vi "2Dstart_BD_ver10_two_daqs.vi"(0 "Master Ctr (Ctr0)":tag, 1 "Master Ctr Terminal (PFI0)":tag, 2 "Galvo Hardware":T2, 3 "Camera Hardware":T1, 4 "input cluster":T4, 5 "error in (no error)":errorcluster, 6 "B-Scan Frequency":dbl=100.0, 7 "A-scans per Image":u32, 8 "Camera Delay (us)":dbl format="%.6f", 9 "A-scans per Cross Section":u32, 11 "Galvo Trigg per Cross Section":u32) -> (13 "Image Size":u32, 14 "Master Ctr Task Out":refnum<k21>, 15 "Galvo AO Task Out":refnum<k21>, 16 "Camera Ctr Task Out":refnum<k21>, 17 "Galvo Ctr Task Out":refnum<k21>, 18 "output cluster for DLL":T3, 19 "AO Err Out":errorcluster)   [LabVIEW 2017]
uses:
  <vilib>/DAQmx/write.llb/DAQmx Write (Analog 2D DBL NChan NSamp).vi
  <vilib>/DAQmx/create/channels.llb/DAQmx Create Channel (CO-Pulse Generation-Frequency).vi
  <vilib>/DAQmx/configure/timing.llb/DAQmx Timing (Implicit).vi
  <vilib>/DAQmx/configure/trigger.llb/DAQmx Start Trigger (Digital Edge).vi
  <vilib>/DAQmx/create/channels.llb/DAQmx Create Channel (AO-Voltage-Basic).vi
  <vilib>/DAQmx/configure/timing.llb/DAQmx Timing (Sample Clock).vi
  <vilib>/DAQmx/miscellaneous.llb/DAQmx Fill In Error Info.vi
  <resource>/objmgr/daqmx.rc
panel:
  out "B-Scan Frequency 2":dbl
  in  "counter":tag
  out "error out":errorcluster
  out "task out":refnum<k21>
  in  "2D frequency":i16
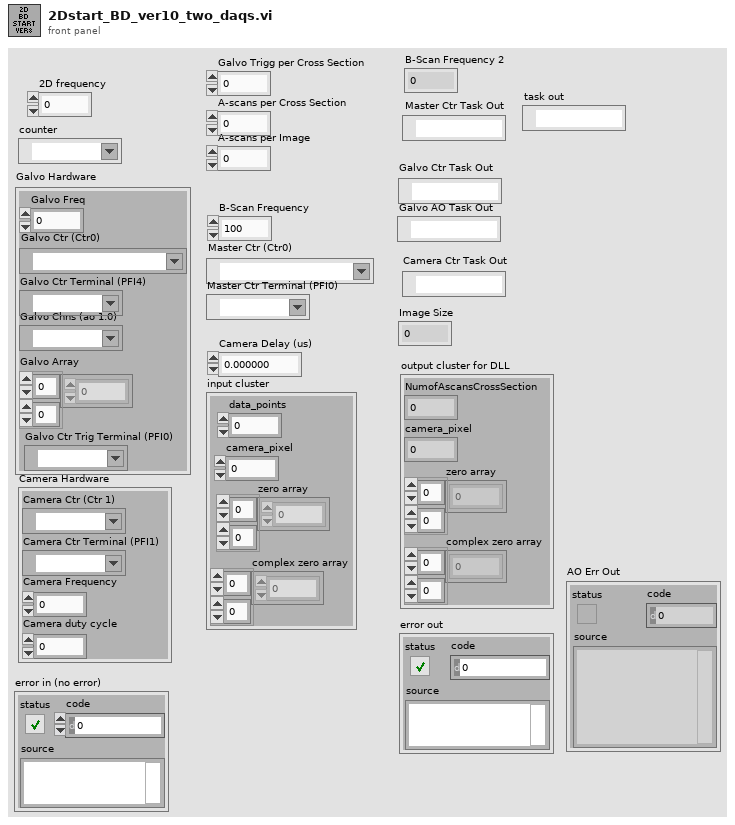
[diagram p1: front panel]
types:
  T1 = cluster{"Camera Ctr (Ctr 1)":tag, "Camera Ctr Terminal (PFI1)":tag, "Camera Frequency":dbl, "Camera duty cycle":dbl}
  T2 = cluster{"Galvo Array":dbl[][], "Galvo Chns (ao 1:0)":tag, "Galvo Ctr (Ctr0)":tag, "Galvo Ctr Terminal (PFI4)":tag, "Galvo Freq":dbl, "Galvo Ctr Trig Terminal (PFI0)":tag}
  T3 = cluster{"NumofAscansCrossSection":i32, "camera_pixel":i32, "zero array":dbl[][], "complex zero array":dbl[][]}
  T4 = cluster{"data_points":i32, "camera_pixel":i32, "zero array":dbl[][], "complex zero array":dbl[][]}
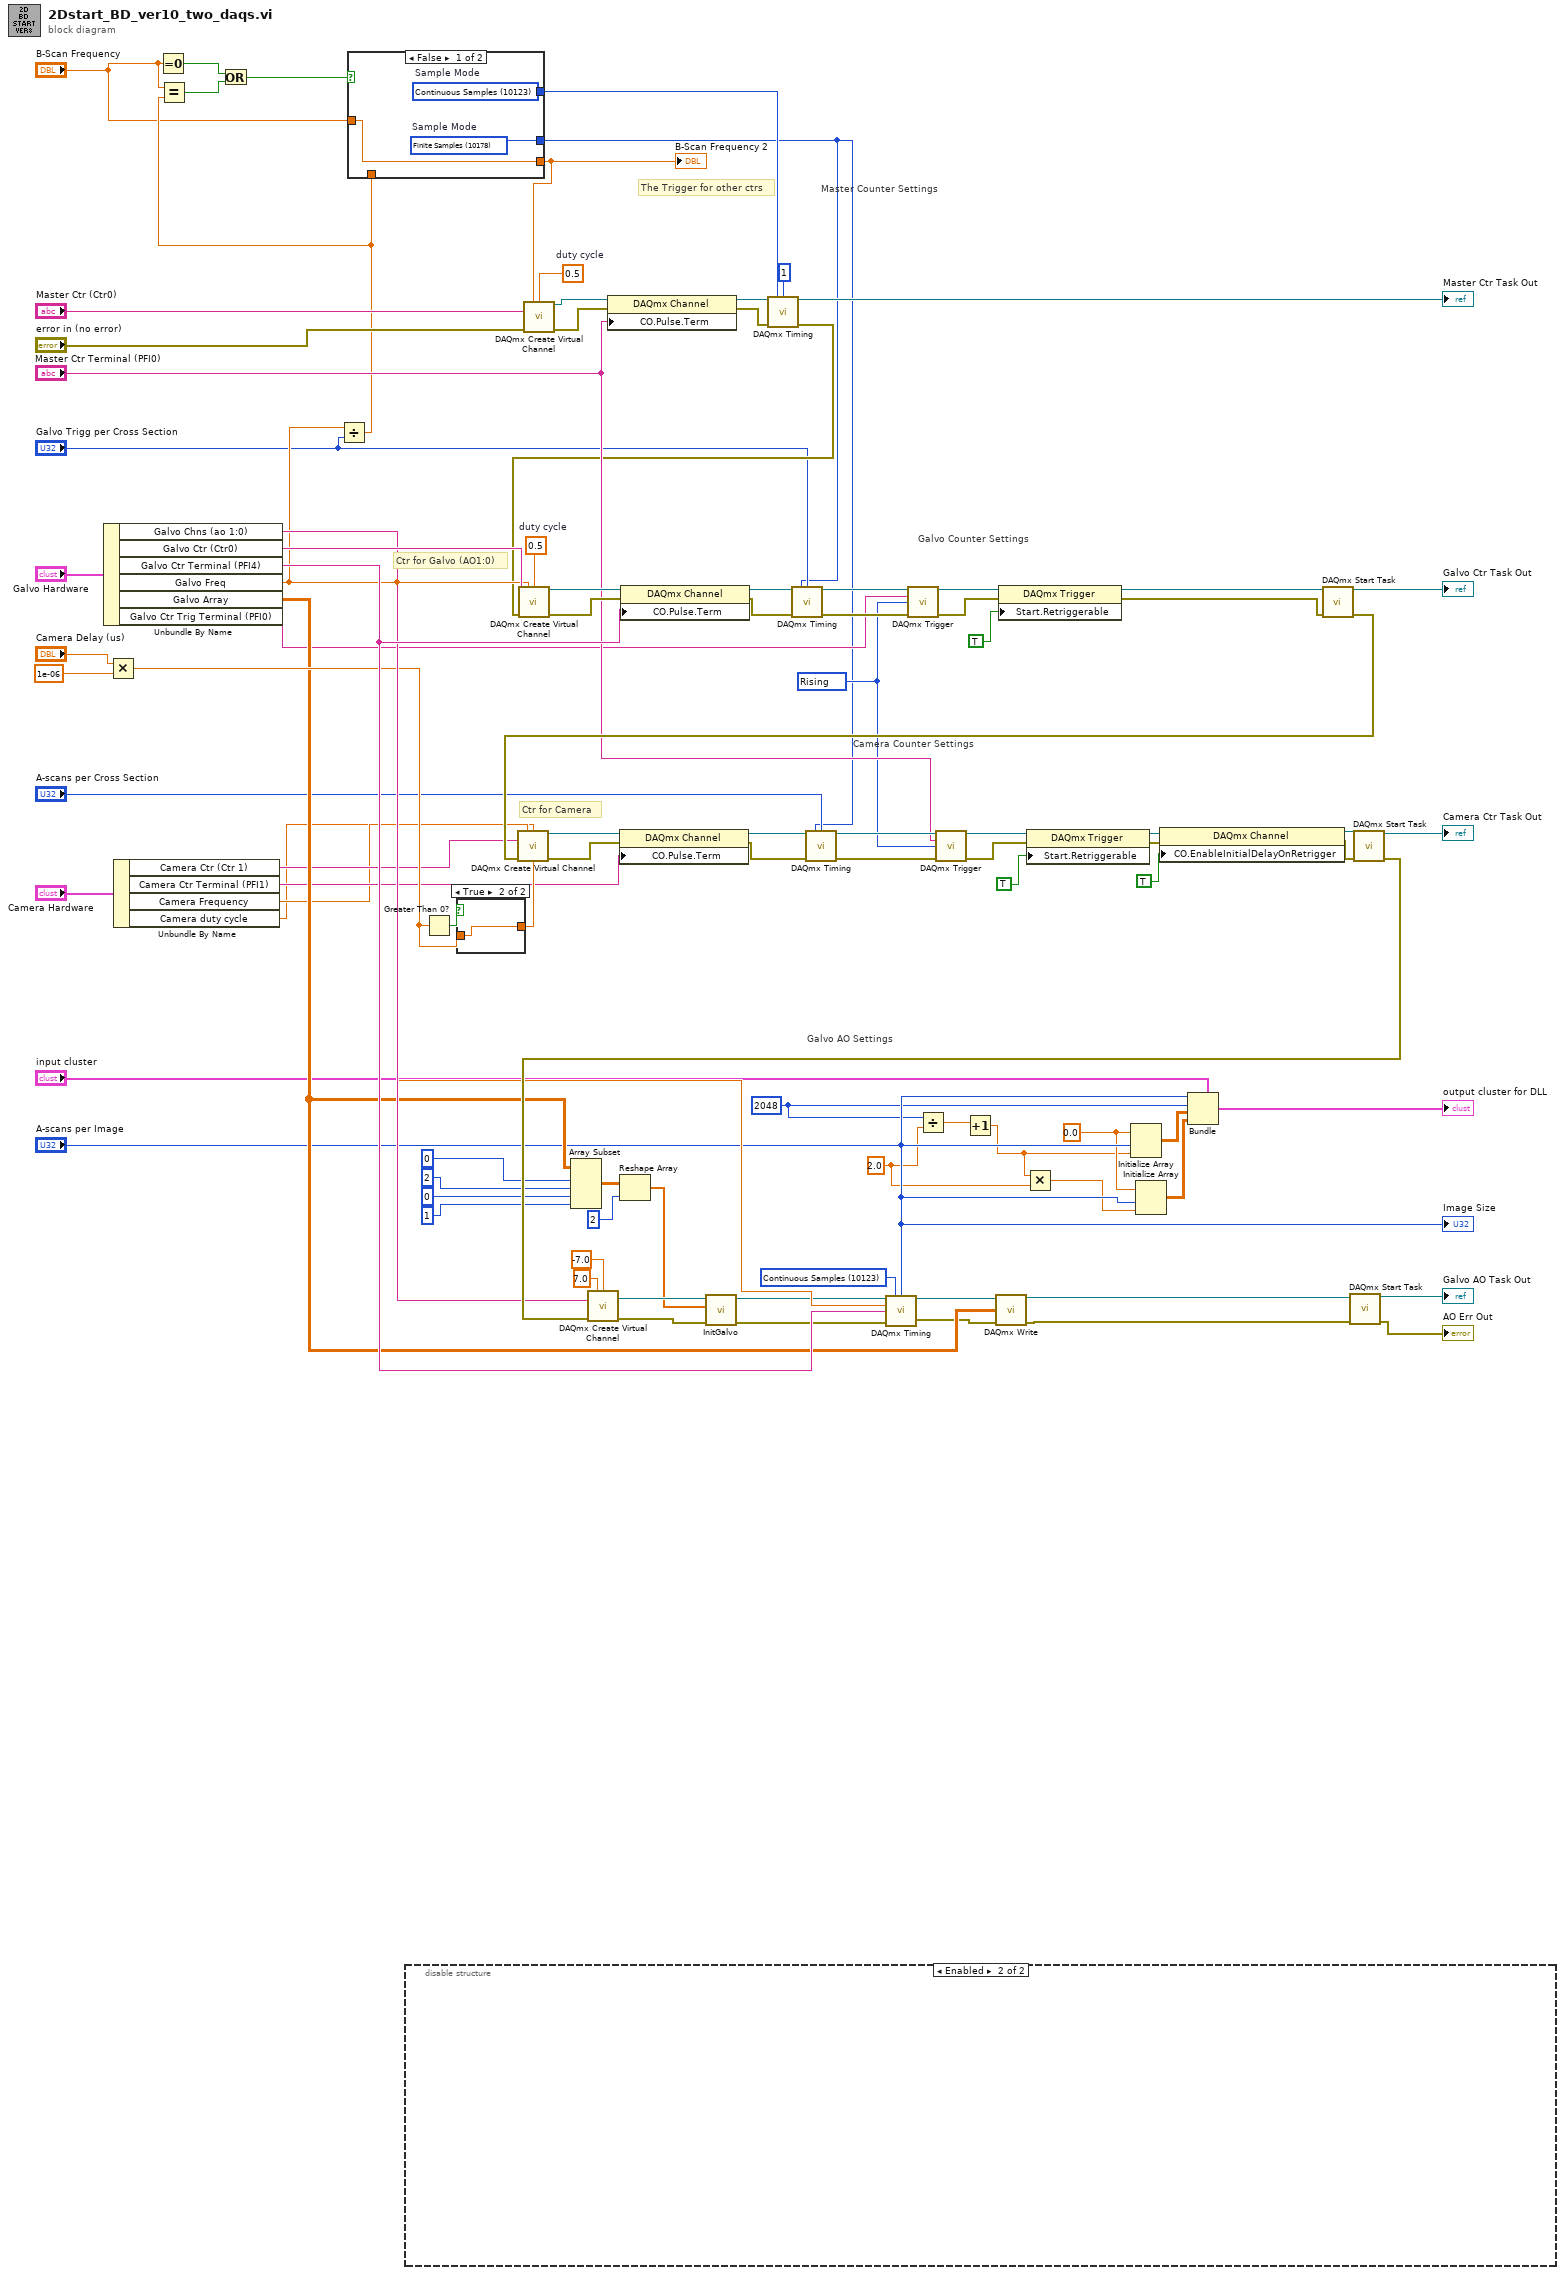
[diagram p0: block diagram]
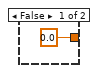
[diagram p2: hidden frame]
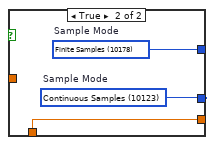
[diagram p3: hidden frame]
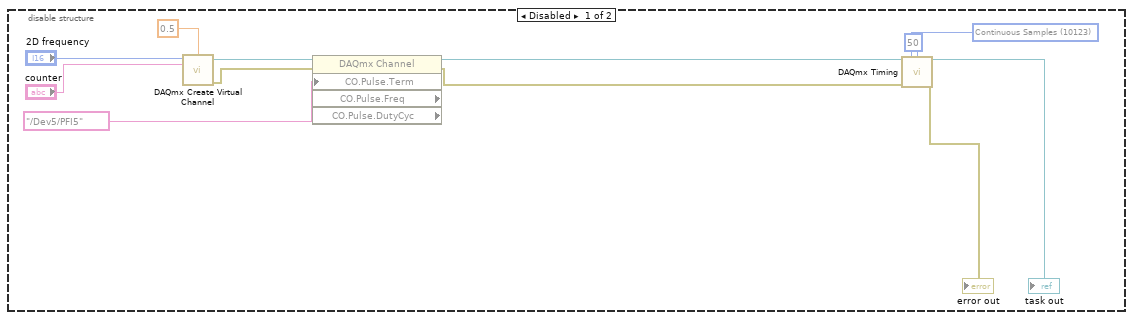
[diagram p4: hidden frame]
diagram:
  w2 = 2048 ("camera_pixel")
  w5 = 2.0 ("y")
  w32 = 0.0 ("element")
  w29 = 10123 items=["Finite Samples"=10178, "Continuous Samples"=10123, "Hardware Timed Single Point"=12522] ("sample mode")
  w50 = 10280 items=["Rising"=10280, "Falling"=10171] ("edge")
  w92 = 0.5  # duty cycle
  w97 = 0.5  # duty cycle
  # "Galvo AO Settings"
  # "Camera Counter Settings"
  # "Galvo Counter Settings"
  # "Master Counter Settings"
  # "Ctr for Camera"
  # "Ctr for Galvo (AO1:0)"
  # "The Trigger for other ctrs"
  n1 = Unbundle By Name("Galvo Hardware") -> ("Galvo Chns (ao 1:0)"=w69:tag, "Galvo Ctr (Ctr0)"=w71:tag, "Galvo Ctr Terminal (PFI4)"=w72:tag, "Galvo Freq"=w61:dbl, "Galvo Array"=w49:dbl[][], "Galvo Ctr Trig Terminal (PFI0)"=w14:tag)
  n2 = Multiply(x="Camera Delay (us)", y=1e-06) -> (x*y=w56:dbl)
  n3 = Unbundle By Name("Camera Hardware") -> ("Camera Ctr (Ctr 1)"=w47:tag, "Camera Ctr Terminal (PFI1)"=w46:tag, "Camera Frequency"=w45:dbl, "Camera duty cycle"=w44:dbl)
  n4 = Equal To 0?(x="B-Scan Frequency") -> (x = 0?=w41:bool)
  n5 = Divide(x=w61, y="Galvo Trigg per Cross Section") -> (x/y=w43:dbl)
  n6 = Equal?(x="B-Scan Frequency", y=w43) -> (x = y?=w40:bool)
  n7 = Or(x=w41, y=w40) -> (x .or. y?=w39:bool)
  n8 = case shown="False" w39 {
    tunnel: "B-Scan Frequency" -> [w103 _]
    tunnel: [w103 w106] -> w53
    tunnel: w43 -> [_ w106]
    tunnel: [w102 w105] -> w52
    tunnel: [w101 w104] -> w1
    frame False {
      w101 = 10178 items=["Finite Samples"=10178, "Continuous Samples"=10123, "Hardware Timed Single Point"=12522]  # Sample Mode
      w102 = 10123 items=["Finite Samples"=10178, "Continuous Samples"=10123, "Hardware Timed Single Point"=12522]  # Sample Mode
    }
    frame True {
      w104 = 10123 items=["Finite Samples"=10178, "Continuous Samples"=10123, "Hardware Timed Single Point"=12522]  # Sample Mode
      w105 = 10178 items=["Finite Samples"=10178, "Continuous Samples"=10123, "Hardware Timed Single Point"=12522]  # Sample Mode
    }
  }
  "B-Scan Frequency 2" <- w53
  n9 = disable-structure shown="Enabled" {
    frame Disabled {
      w115 = 10123 items=["Finite Samples"=10178, "Continuous Samples"=10123, "Hardware Timed Single Point"=12522] ("sample mode")
      n10 = call-poly <vilib>:"DAQmx Create Virtual Channel.vi"("frequency"="2D frequency", "duty cycle"=0.5, "counter"="counter") -> ("task out"=w111:refnum<k21>, "error out"=w110:errorcluster)  [unwired: 6 in, 5 out]
      n11 = property class="DAQmx Channel" props=["CO.Pulse.Term", "CO.Pulse.Freq", "CO.Pulse.DutyCyc"](reference=w111, error in=w110, "CO.Pulse.Term"=tag "/Dev5/PFI5") -> (reference out=w109:refnum<k21>, error out=w108:errorcluster)  [unwired: 2 out]
      n12 = call-poly <vilib>:"DAQmx Timing.vi"("task/channels in"=w109, "sample mode"=w115, "samples per channel"=50, "error in"=w108) -> ("task out"=→"task out":refnum<k21>, "error out"=→"error out":errorcluster)  [unwired: 2 in, 8 out]
    }
    frame Enabled {
    }
  }
  n13 = Greater Than 0?(x=w56) -> (x > 0?=w60:bool)
  n14 = case shown="True" w60 {
    tunnel: w56 -> [_ w120]
    tunnel: [0.0 ("Camera Delay") w120] -> w59
    frame False {
    }
    frame True {
    }
  }
  n15 = call-poly <vilib>:"DAQmx Create Virtual Channel.vi"("frequency"=w53, "duty cycle"=w97, "counter"="Master Ctr (Ctr0)", "error in"="error in (no error)") -> ("task out"=w100:refnum<k21>, "error out"=w99:errorcluster)  [unwired: 10 in]
  n16 = Array Subset(array=w49, index (row)=0 ("index"), length (row)=2 ("length"), index (col)=0 ("index"), length (col)=1 ("length")) -> (w24:dbl[][])
  n17 = property class="DAQmx Channel"(reference=w100, error in=w99, "CO.Pulse.Term"="Master Ctr Terminal (PFI0)") -> (reference out=w96:refnum<k21>, error out=w95:errorcluster)
  n18 = Reshape Array(w24, 2 ("dimension size")) -> (w19:dbl[])
  n19 = call-poly <vilib>:"DAQmx Timing.vi"("task/channels in"=w96, "sample mode"=w52, "samples per channel"=1, "error in"=w95) -> ("task out"=→"Master Ctr Task Out":refnum<k21>, "error out"=w55:errorcluster)  [unwired: 10 in]
  n20 = call-poly <vilib>:"DAQmx Create Virtual Channel.vi"("frequency"=w61, "duty cycle"=w92, "counter"=w71, "error in"=w55) -> ("task out"=w94:refnum<k21>, "error out"=w93:errorcluster)  [unwired: 10 in]
  n21 = property class="DAQmx Channel"(reference=w94, error in=w93, "CO.Pulse.Term"=w72) -> (reference out=w81:refnum<k21>, error out=w80:errorcluster)
  n22 = call-poly <vilib>:"DAQmx Timing.vi"("task/channels in"=w81, "sample mode"=w1, "samples per channel"="Galvo Trigg per Cross Section", "error in"=w80) -> ("task out"=w79:refnum<k21>, "error out"=w78:errorcluster)  [unwired: 10 in]
  n23 = call-poly <vilib>:"DAQmx Trigger.vi"("task/channels in"=w79, "source"=w14, "edge"=w50, "error in"=w78) -> ("task out"=w90:refnum<k21>, "error out"=w91:errorcluster)  [unwired: 10 in]
  n24 = Divide(x=w2, y=w5) -> (x/y=w6:dbl)
  n25 = Increment(x=w6) -> (x+1=w4:dbl)
  n26 = property class="DAQmx Trigger"(reference=w90, error in=w91, "Start.Retriggerable"=TRUE) -> (reference out=w13:refnum<k21>, error out=w12:errorcluster)
  n27 = Multiply(x=w4, y=w5) -> (x*y=w3:dbl)
  n28 = Initialize Array(w32, "A-scans per Image", w4) -> (w30:dbl[][])
  n29 = Initialize Array(w32, "A-scans per Image", w3) -> (w31:dbl[][])
  n30 = Bundle(cluster="input cluster", "data_points"="A-scans per Image", "camera_pixel"=w2, "zero array"=w30, "complex zero array"=w31) -> (→"output cluster for DLL":T4)
  n31 = call <vilib>:"DAQmx Start Task.vi"("task/channels in"=w13, "error in"=w12) -> ("task out"=→"Galvo Ctr Task Out":refnum<k21>, "error out"=w73:errorcluster)  [unwired: 12 in]
  n32 = call-poly <vilib>:"DAQmx Create Virtual Channel.vi"("frequency"=w45, "duty cycle"=w44, "counter"=w47, "error in"=w73, "initial delay"=w59) -> ("task out"=w87:refnum<k21>, "error out"=w86:errorcluster)  [unwired: 9 in]
  n33 = property class="DAQmx Channel"(reference=w87, error in=w86, "CO.Pulse.Term"=w46) -> (reference out=w77:refnum<k21>, error out=w76:errorcluster)
  n34 = call-poly <vilib>:"DAQmx Timing.vi"("task/channels in"=w77, "sample mode"=w1, "samples per channel"="A-scans per Cross Section", "error in"=w76) -> ("task out"=w75:refnum<k21>, "error out"=w74:errorcluster)  [unwired: 10 in]
  n35 = call-poly <vilib>:"DAQmx Trigger.vi"("task/channels in"=w75, "source"="Master Ctr Terminal (PFI0)", "edge"=w50, "error in"=w74) -> ("task out"=w84:refnum<k21>, "error out"=w85:errorcluster)  [unwired: 10 in]
  n36 = property class="DAQmx Trigger"(reference=w84, error in=w85, "Start.Retriggerable"=TRUE) -> (reference out=w67:refnum<k21>, error out=w66:errorcluster)
  n37 = property class="DAQmx Channel"(reference=w67, error in=w66, "CO.EnableInitialDelayOnRetrigger"=TRUE) -> (reference out=w64:refnum<k21>, error out=w63:errorcluster)
  n38 = call <vilib>:"DAQmx Start Task.vi"("task/channels in"=w64, "error in"=w63) -> ("task out"=→"Camera Ctr Task Out":refnum<k21>, "error out"=w70:errorcluster)  [unwired: 12 in]
  n39 = call-poly <vilib>:"DAQmx Create Virtual Channel.vi"("maximum value"=7.0, "minimum value"=-7.0, "physical channels"=w69, "error in"=w70) -> ("task out"=w20:refnum<k21>, "error out"=w23:errorcluster)  [unwired: 5 in, 5 out]
  n40 = call "InitGalvo.vi"("error in"=w23, "Output Array"=w19, "task/channels in"=w20) -> ("error out"=w22:errorcluster, "task out"=w21:refnum<k21>)  [unwired: 7 in]
  n41 = call-poly <vilib>:"DAQmx Timing.vi"("task/channels in"=w21, "sample mode"=w29, "samples per channel"="A-scans per Image", "rate"=w61, "source"=w72, "error in"=w22) -> ("task out"=w28:refnum<k21>, "error out"=w33:errorcluster)  [unwired: 1 in, 7 out]
  n42 = call-poly <vilib>:"DAQmx Write.vi"("task/channels in"=w28, "data"=w49, "error in"=w33) -> ("task out"=w11:refnum<k21>, "error out"=w10:errorcluster)  [unwired: 1 in, 10 out]
  n43 = call <vilib>:"DAQmx Start Task.vi"("task/channels in"=w11, "error in"=w10) -> ("task out"=→"Galvo AO Task Out":refnum<k21>, "error out"=→"AO Err Out":errorcluster)  [unwired: 12 in]
  "Image Size" <- "A-scans per Image"
